vi "SaveVector.vi"(10 "error in (no error)":errorcluster, 11 "Leap Vector":refnum<k24>) -> (2 "error out":errorcluster, 3 "Vector":T1={"Pitch"=nan, "Yaw"=nan, "Roll"=nan, "Magnitude"=nan, "XYZ"=[nan, nan, nan]})   [LabVIEW 2011, in "LVH-Leap.lvlib"]
uses:
  LVH-Leap.lvlib
  C:/github/labviewhacker/LVH-Leap/LabVIEW/vi.lib/LabVIEW Hacker/Leap/Private/Libs/LeapCSharp.NET3.5.dll
  Libs/LeapCSharp.NET3.5.dll
  Type Defs/Vector.ctl
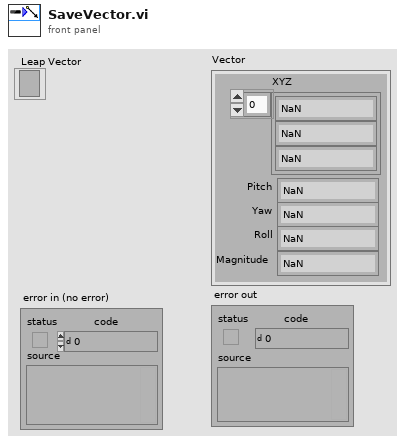
[diagram p1: front panel]
types:
  T1 = typedef "LVH-Leap.lvlib/Vector.ctl" = cluster{"Pitch":sgl, "Yaw":sgl, "Roll":sgl, "Magnitude":sgl, "XYZ":sgl[]}
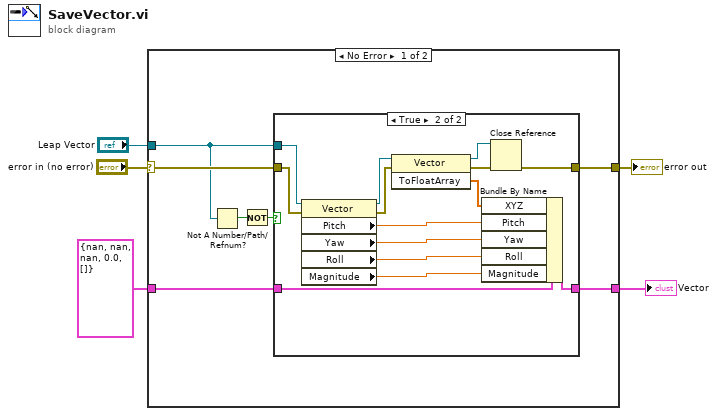
[diagram p0: block diagram]
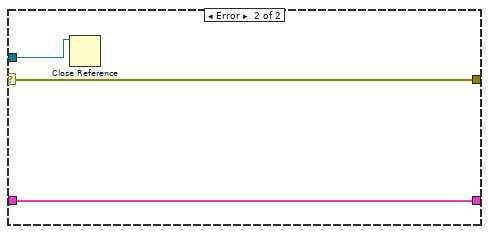
[diagram p3: hidden frame]
diagram:
  n1 = case shown="No Error" "error in (no error)" {
    selector: "error in (no error)" -> [w11 w30]
    tunnel: "Leap Vector" -> [w8 w29]
    tunnel: [w12 w31] -> w4
    tunnel: [w10 w30] -> w2
    tunnel: T1 {"Pitch"=nan, "Yaw"=nan, "Roll"=nan, "Magnitude"=0.0, "XYZ"=[]} ("Vector") -> [w9 w31]
    frame No Error {
      n2 = Not A Number/Path/Refnum?(number/path/refnum=w8) -> (NaN/Path/Refnum?=w6:bool)
      n3 = Not(x=w6) -> (.not. x?=w7:bool)
      n4 = case shown="True" w7 {
        tunnel: w9 -> [w14 w28]
        tunnel: [w13 w27] -> w10
        tunnel: [w14 w26] -> w12
        tunnel: w11 -> [w13 w24]
        tunnel: w8 -> [_ w25]
        frame False {
        }
        frame True {
          n5 = property class="Vector"(reference=w25, error in=w24) -> (reference out=w18:refnum<k24>, error out=w19:errorcluster, "Pitch"=w23:sgl, "Yaw"=w22:sgl, "Roll"=w21:sgl, "Magnitude"=w20:sgl)
          n6 = invoke class="Vector" method="ToFloatArray"(reference=w18, error in=w19) -> (reference out=w15:refnum<k24>, error out=w16:errorcluster, "ToFloatArray"=w17:sgl[])  [unwired: 1 in]
          n7 = Bundle By Name(cluster=w28, "XYZ"=w17, "Pitch"=w23, "Yaw"=w22, "Roll"=w21, "Magnitude"=w20) -> (w26:T1)
          n8 = Close Reference(reference=w15, error in (no error)=w16) -> (error out=w27:errorcluster)
        }
      }
    }
    frame Error {
      n9 = Close Reference(reference=w29) -> ()  [unwired: 1 in, 1 out]
    }
  }
  "Vector" <- w4
  "error out" <- w2
